vi "stop.vi"(8 "error in (no error)":errorcluster, 11 "ILC in":refnum<class "ILC.lvclass">) -> (0 "error out":errorcluster, 3 "ILC out":refnum<class "ILC.lvclass">)   [LabVIEW 2013, in "ILCCommon.lvlib" / "ILC.lvclass"]
uses:
  <userlib>/Common/ILC/ILC/ILC.lvclass
  <userlib>/Common/ILC/ILC/ILC.lvclass/ILC.ctl
  <userlib>/Common/SerialProtocols/SerialCommunicator/SerialCommunicator.lvclass
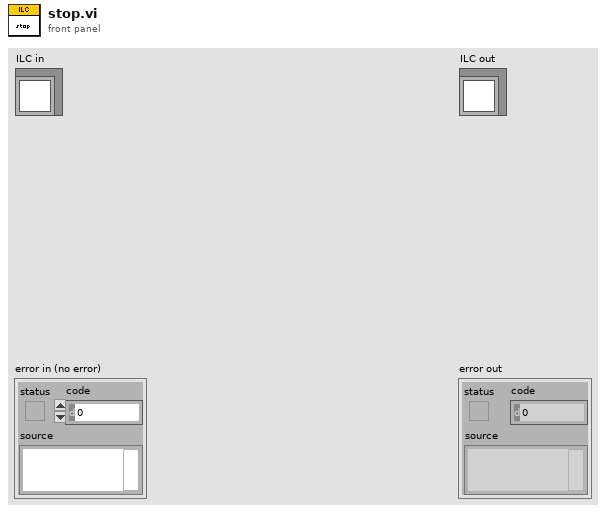
[diagram p1: front panel]
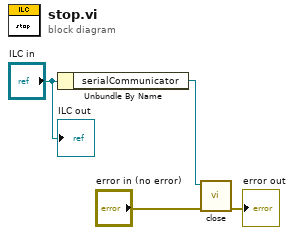
[diagram p0: block diagram]
diagram:
  n1 = Unbundle By Name("ILC in") -> ("serialCommunicator"=w3:refnum<class "SerialCommunicator.lvclass">)
  n2 = call-dynamic "close.vi"("error in (no error)"="error in (no error)", "SerialCommunicator in"=w3) -> ("error out"=→"error out":errorcluster)  [unwired: 8 in, 1 out]
  "ILC out" <- "ILC in"
